vi "F05 Config Parameter.vi"(4 "error in (no error)":errorcluster, 5 "参数值":dbl=50.0, 6 "参数类型":T1(ring), 7 "MyIndex":u8) -> (0 "error out":errorcluster, 1 "Pass/Fail":bool)   [LabVIEW 2015]
uses:
  <vilib>/Instr/_visa.llb/VISA Configure Serial Port (Instr).vi
panel:
  out "VISA":refnum<visa-resource-name> caption="VISA资源名称输出"
  out "write string":string
  # "Config the duty cycle of Waveform"
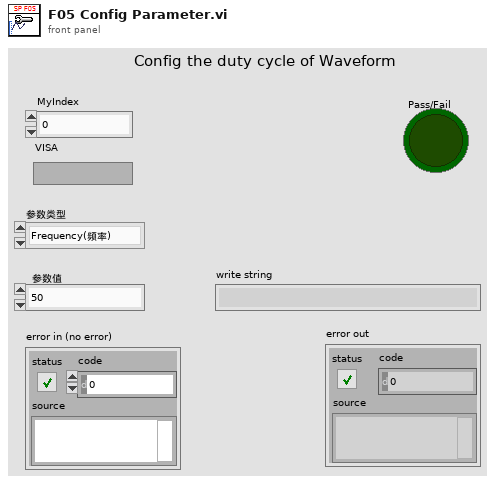
[diagram p1: front panel]
types:
  T1 = enum16{"Frequency(频率)", "Ａmplitude(幅度)", "Voltage offset(电压偏置) ", "Duty Cycle(占空比)"}
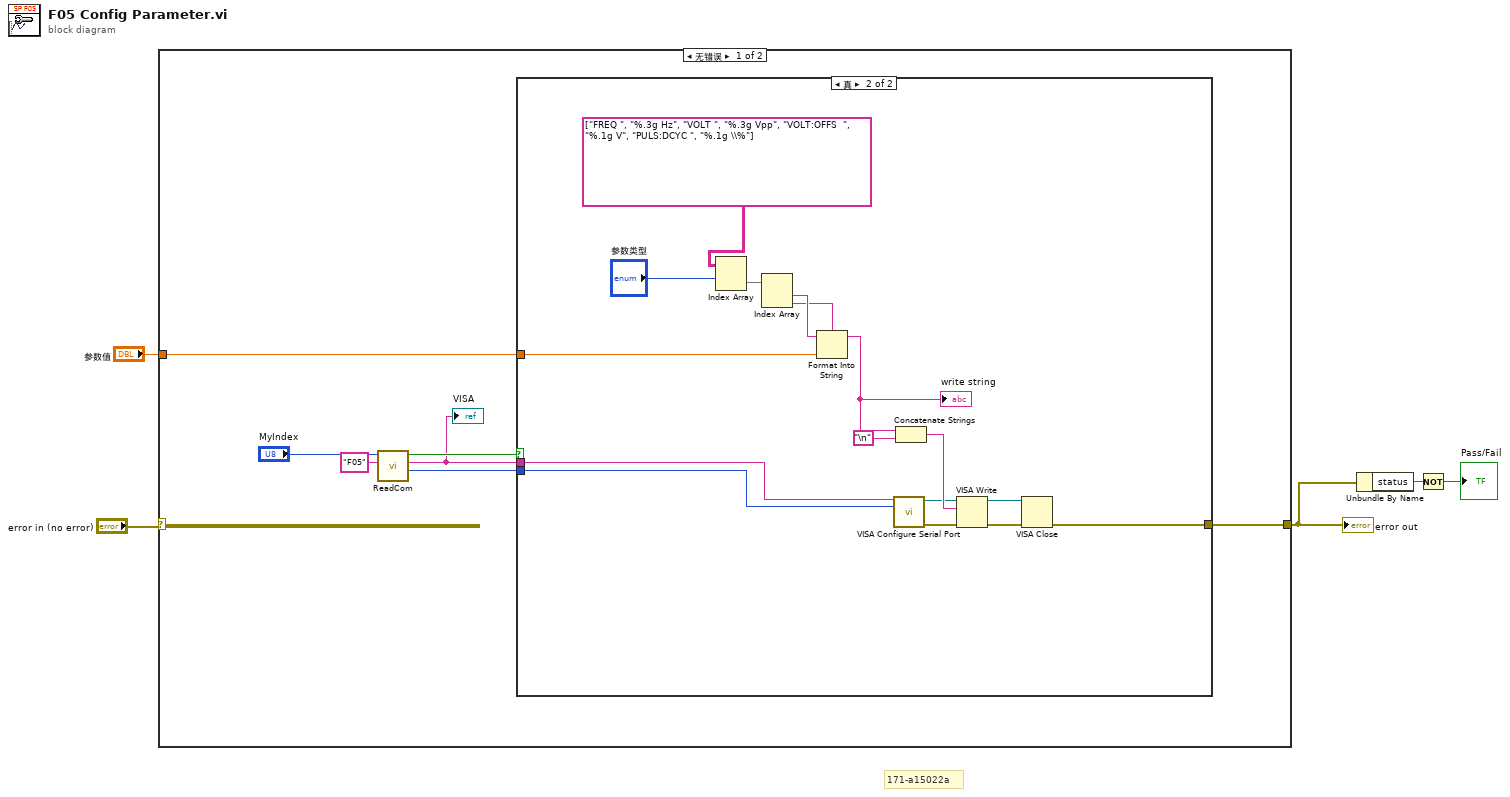
[diagram p0: block diagram]
diagram:
  # "171-a15022a"
  n1 = case shown="无错误" "error in (no error)" {
    selector: "error in (no error)" -> [_ w29]
    tunnel: [w11 w29] -> w1
    tunnel: "参数值" -> [w12 _]
    frame No Error {
      n2 = call "ReadCom.vi"("仪器名称"="F05", "MyIndex"="MyIndex") -> ("Baudrate"=w6:i32, "COM"=w7:string, "OK?"=w8:bool)  [unwired: 7 in]
      "VISA" <- w7
      n3 = case shown="真" w8 {
        tunnel: w12 -> [_ w25]
        tunnel: [_ w23] -> w11
        tunnel: w7 -> [_ w14]
        tunnel: w6 -> [_ w13]
        frame False {
        }
        frame True {
          n4 = Index Array(array=string[][] [["FREQ ", "%.3g Hz"], ["VOLT ", "%.3g Vpp"], ["VOLT:OFFS  ", "%.1g V"], ["PULS:DCYC ", "%.1g \\%"]], index (row)="参数类型") -> (element=w18:string[])  [unwired: 1 in]
          n5 = Index Array(array=w18) -> (element #1=w17:string, element #2=w16:string)  [unwired: 2 in]
          n6 = Format Into String(format string=w16, initial string=w17, w25) -> (resulting string=w28:string)  [unwired: 1 in, 1 out]
          "write string" <- w28
          n7 = call-poly "VISA Configure Serial Port"("VISA resource name"=w14, "baud rate (9600)"=w13) -> ("VISA resource name out"=w20:refnum<visa-resource-name>, "error out"=w24:errorcluster)  [unwired: 12 in]
          n8 = Concatenate Strings(w28, "\n") -> (w26:string)
          n9 = VISA Write(VISA resource name=w20, write buffer=w26, error in (no error)=w24) -> (VISA resource name out=w21:refnum<visa-resource-name>, error out=w22:errorcluster)  [unwired: 1 out]
          n10 = VISA Close(VISA resource name=w21, error in (no error)=w22) -> (error out=w23:errorcluster)
        }
      }
    }
    frame Error {
    }
  }
  "error out" <- w1
  n11 = Unbundle By Name(w1) -> ("status"=w3:bool)
  n12 = Not(x=w3) -> (.not. x?=→"Pass/Fail":bool)
